vi "Current Measurement.vi"(0 "Cature Load Currrent Pin Name":string, 1 "Load Current Sequence":dbl[](array[numeric]), 2 "Current Measurement Option":T1, 5 "Total Aquisition Time (s)":dbl, 7 "Shunt Resistance":dbl, 9 "Measured Scope Load Current":cluster{"x-axis":dbl[], "wfm":dbl[]}, 11 "error in (no error)":errorcluster, 12 "Trigger Delay":dbl) -> (4 "Measured Load Current":cluster{"x-axis":dbl[], "wfm":dbl[]}, 15 "error out":errorcluster)   [LabVIEW 2020, in "LDO Load Transient.lvlib"]
uses:
  LDO Load Transient.lvlib
  Typedefs/Current Measurement Type.ctl
  90de16d1-2031-466e-9767-c62d8a014f4c.vi
  <userlib>/_Soliton/Measurement Suite/Reusables/InstrumentSessionAPIs/SessionManagerApiPath.vi
  <vilib>/Utility/sysdir.llb/Get System Directory.vi
  <vilib>/Utility/LVLibp/Get Exported File Path.vi
  <userlib>/_Soliton/Measurement Suite/Reusables/Errors/Error 6001.vi
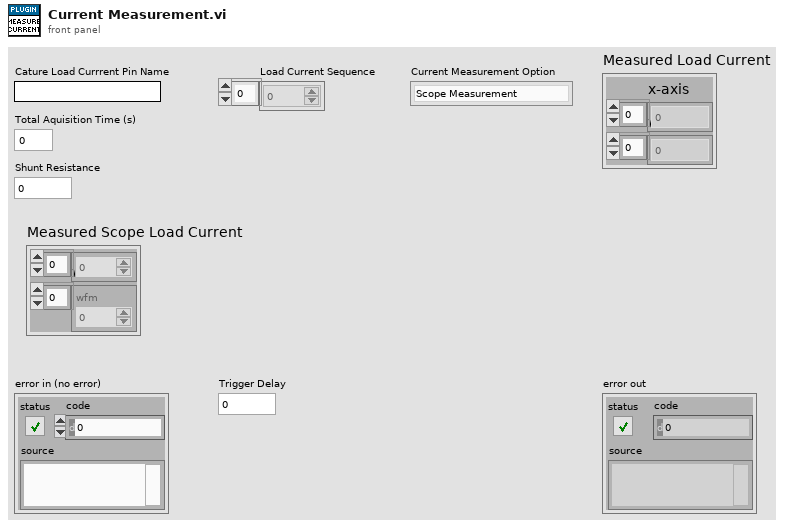
[diagram p1: front panel]
types:
  T1 = typedef "LDO Load Transient.lvlib/Current Measurement Type.ctl" = enum16{"Scope Measurement", "SMU Measurement"}
  T2 = cluster{"relativeInitialX":dbl, "xIncrement":dbl, "wfm":dbl[]}
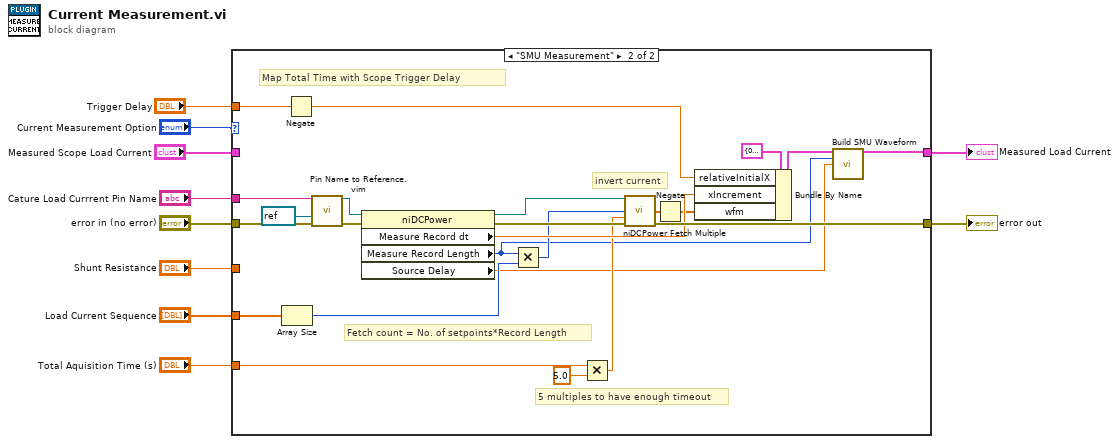
[diagram p0: block diagram]
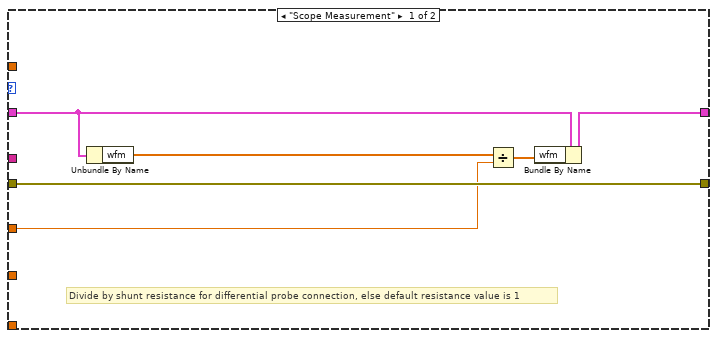
[diagram p2: hidden frame]
diagram:
  n1 = case shown="\"SMU Measurement\"" "Current Measurement Option" {
    tunnel: [w15 w17] -> w10
    tunnel: [w16 w38] -> w9
    tunnel: "error in (no error)" -> [w16 w37]
    tunnel: "Cature Load Currrent Pin Name" -> [_ w36]
    tunnel: "Shunt Resistance" -> [w14 _]
    tunnel: "Total Aquisition Time (s)" -> [_ w26]
    tunnel: "Load Current Sequence" -> [_ w29]
    tunnel: "Trigger Delay" -> [_ w22]
    tunnel: "Measured Scope Load Current" -> [w11 _]
    frame "Scope Measurement" {
      # "Divide by shunt resistance for differential probe connection, else default resistance value is 1"
      n2 = Unbundle By Name(w11) -> ("wfm"=w12:dbl[])
      n3 = Divide(x=w12, y=w14) -> (x/y=w13:dbl[])
      n4 = Bundle By Name(cluster=w11, "wfm"=w13) -> (w15:cluster{"x-axis":dbl[], "wfm":dbl[]})
    }
    frame "SMU Measurement" {
      # "invert current"
      # "5 multiples to have enough timeout"
      # "Fetch count = No. of setpoints*Record Length"
      # "Map Total Time with Scope Trigger Delay"
      n5 = Array Size(array=w29) -> (size(s)=w28:i32)
      n6 = Negate(x=w22) -> (-x=w21:dbl)
      n7 = call "Pin Name to Reference.vim"("Pin Name"=w36, "type"=refnum<k15> refnum ("instrument handle"), "error in (no error)"=w37) -> ("Reference"=w32:refnum<k15>, "error out"=w39:errorcluster)  [unwired: 7 in, 4 out]
      n8 = property class="niDCPower"(reference=w32, error in=w39) -> (reference out=w31:refnum<k15>, error out=w33:errorcluster, "Measure Record dt"=w30:dbl, "Measure Record Length"=w19:i32, "Source Delay"=w18:dbl)
      n9 = Multiply(x=w19, y=w28) -> (x*y=w27:i32)
      n10 = Multiply(x=w26, y=5.0) -> (x*y=w24:dbl)
      n11 = call <instrlib>:"niDCPower Fetch Multiple.vi"("instrument handle"=w31, "count (1)"=w27, "timeout (sec)"=w24, "error in (no error)"=w33) -> ("current measurements"=w34:dbl[], "error out"=w38:errorcluster)  [unwired: 6 in, 4 out]
      n12 = Negate(x=w34) -> (-x=w23:dbl[])
      n13 = Bundle By Name(cluster=T2 {"relativeInitialX"=0.0, "xIncrement"=0.0, "wfm"=[]}, "relativeInitialX"=w21, "xIncrement"=w30, "wfm"=w23) -> (w20:T2)
      n14 = call "Build SMU Waveform.vi"("Measure Load Current"=w20, "Record Length"=w19, "Source Delay"=w18) -> ("SMU Waveform"=w17:cluster{dbl[], dbl[]})  [unwired: 12 in]
    }
  }
  "Measured Load Current" <- w10
  "error out" <- w9
